vi "ShapekoGlobal.vi"() -> ()   [LabVIEW 2023]
panel:
  out "abort":bool
  out "running?":bool
  out "unlocked":bool
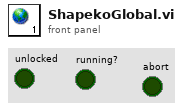
[diagram p1: front panel]
diagram:
